vi "__uintGetTimeout.vi"(8 "Error in (no error)":errorcluster, 11 "UintClass in":refnum<class "UintClass.lvclass">) -> (0 "Error out":errorcluster, 2 "Timeout (-1)":T1=-1, 3 "UintClass out":refnum<class "UintClass.lvclass">)   [LabVIEW 2011, in "UintClass.lvclass"]
uses:
  UintClass.lvclass
  timeout.ctl
  UintClass.lvclass/UintClass.ctl
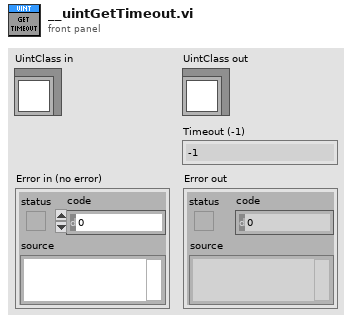
[diagram p1: front panel]
types:
  T1 = typedef "UintClass.lvclass/timeout.ctl" = i32
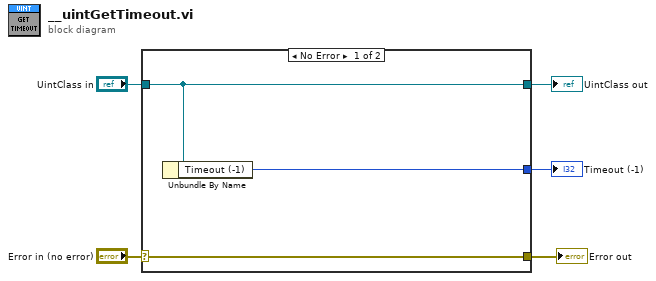
[diagram p0: block diagram]
diagram:
  n1 = case shown="No Error" "Error in (no error)" {
    selector: "Error in (no error)" -> [w8 w9]
    tunnel: [w8 w9] -> w2
    tunnel: [w7 w10] -> w4
    tunnel: "UintClass in" -> [w7 w10]
    tunnel: [w6 _] -> w3
    frame No Error {
      n2 = Unbundle By Name(w7) -> ("Timeout (-1)"=w6:T1)
    }
    frame Error {
    }
  }
  "UintClass out" <- w4
  "Timeout (-1)" <- w3
  "Error out" <- w2
